vi "uTransport_Destroy.vi"(8 "error in (no error)":errorcluster, 11 "uTransport_Event in":refnum<class "uTransport_Event.lvclass">) -> (0 "error out":errorcluster)   [LabVIEW 2023, in "uFramework.lvlib" / "uTransport_Event.lvclass"]
doc: "Do not destroy the event except after the listener loop has stopped. Wire in the error coming out of the loop to the input of this method."
uses:
  uTransport_Event.lvclass
  uTransport_Event.lvclass/uTransport_Event.ctl
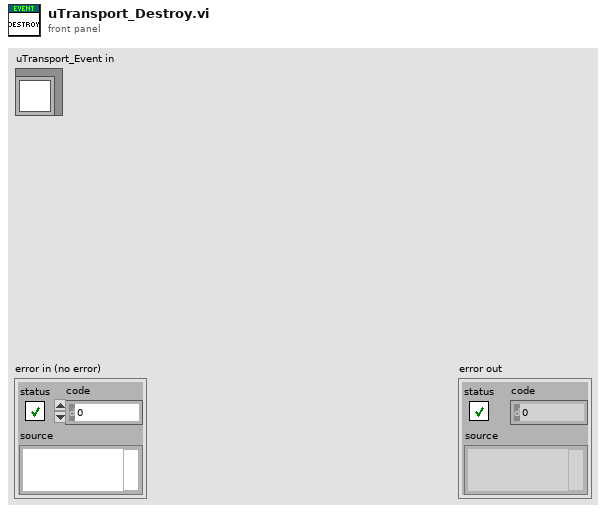
[diagram p1: front panel]
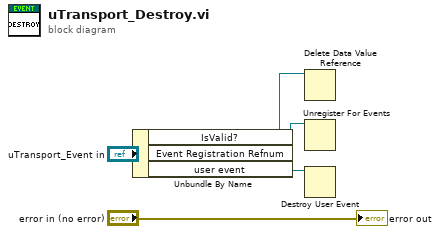
[diagram p0: block diagram]
diagram:
  n1 = Unbundle By Name("uTransport_Event in") -> ("IsValid?"=w1:refnum<data-value>, "Event Registration Refnum"=w3:refnum<event-registration>, "user event"=w5:refnum<user-event>)
  n2 = Delete Data Value Reference(data value reference=w1) -> ()  [unwired: 1 in, 2 out]
  n3 = Unregister For Events(event registration refnum=w3) -> ()  [unwired: 1 in, 1 out]
  n4 = Destroy User Event(user event=w5) -> ()  [unwired: 1 in, 1 out]
  "error out" <- "error in (no error)"
